vi "GenerateCode.vi"(0 "XRef":T10, 1 "Terms":T7, 2 "Diagram":T6, 3 "State In":T1) -> (14 "Generated Code?":T5, 15 "Reply":T3, 16 "Fatal Error Out":T2, 17 "State Out":T1)   [LabVIEW 2015, in "Set Object Parameters.xnode"]
uses:
  Set Object Parameters.xnode
  <vilib>/XNodeSupport/XNodeXNodeRef.ctl
  <vilib>/XNodeSupport/XNodeTermIDPairs.ctl
  <vilib>/XNodeSupport/XNodeTermIDPair.ctl
  <vilib>/XNodeSupport/XNodeTermRef.ctl
  <vilib>/XNodeSupport/XNodeString.ctl
  <vilib>/XNodeSupport/XNodeTopLevelDiagramRef.ctl
  State.ctl
  <vilib>/XNodeSupport/XNodeBool.ctl
  <vilib>/XNodeSupport/XNodeStringArray.ctl
  <vilib>/XNodeSupport/XNodeErrorCluster.ctl
  <vilib>/Utility/miscctls.llb/LVPointTypeDef.ctl
  Insert Key Value Pair.vi
  <vilib>/XNodeSupport/NI_XNodeSupport.lvlib
  JSON Object.lvclass
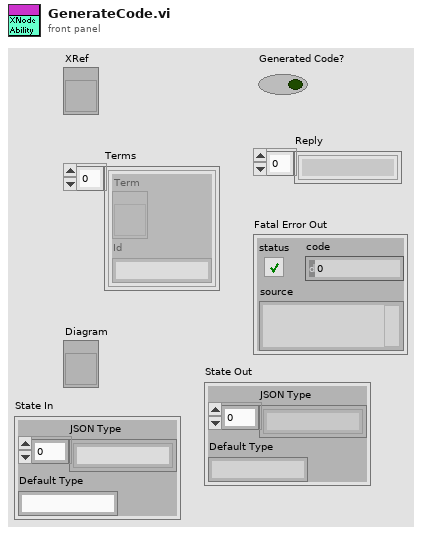
[diagram p1: front panel]
types:
  T1 = typedef "Set Object Parameters.xnode/State.ctl" = cluster{"JSON Type":string[], "Default Type":string}
  T2 = typedef "NI_XNodeSupport.lvlib/XNodeErrorCluster.ctl" = errorcluster
  T3 = typedef "NI_XNodeSupport.lvlib/XNodeStringArray.ctl" = T4[]
  T4 = typedef "NI_XNodeSupport.lvlib/XNodeString.ctl" = string
  T5 = typedef "NI_XNodeSupport.lvlib/XNodeBool.ctl" = bool
  T6 = typedef "NI_XNodeSupport.lvlib/XNodeTopLevelDiagramRef.ctl" = refnum<vi>
  T7 = typedef "NI_XNodeSupport.lvlib/XNodeTermIDPairs.ctl" = T8[]
  T8 = typedef "NI_XNodeSupport.lvlib/XNodeTermIDPair.ctl" = cluster{"Term":T9, "Id":T4}
  T9 = typedef "NI_XNodeSupport.lvlib/XNodeTermRef.ctl" = refnum<vi>
  T10 = typedef "NI_XNodeSupport.lvlib/XNodeXNodeRef.ctl" = refnum<vi>
  T11 = typedef "LVPointTypeDef.ctl" = cluster{"Horizontal":i16, "Vertical":i16}
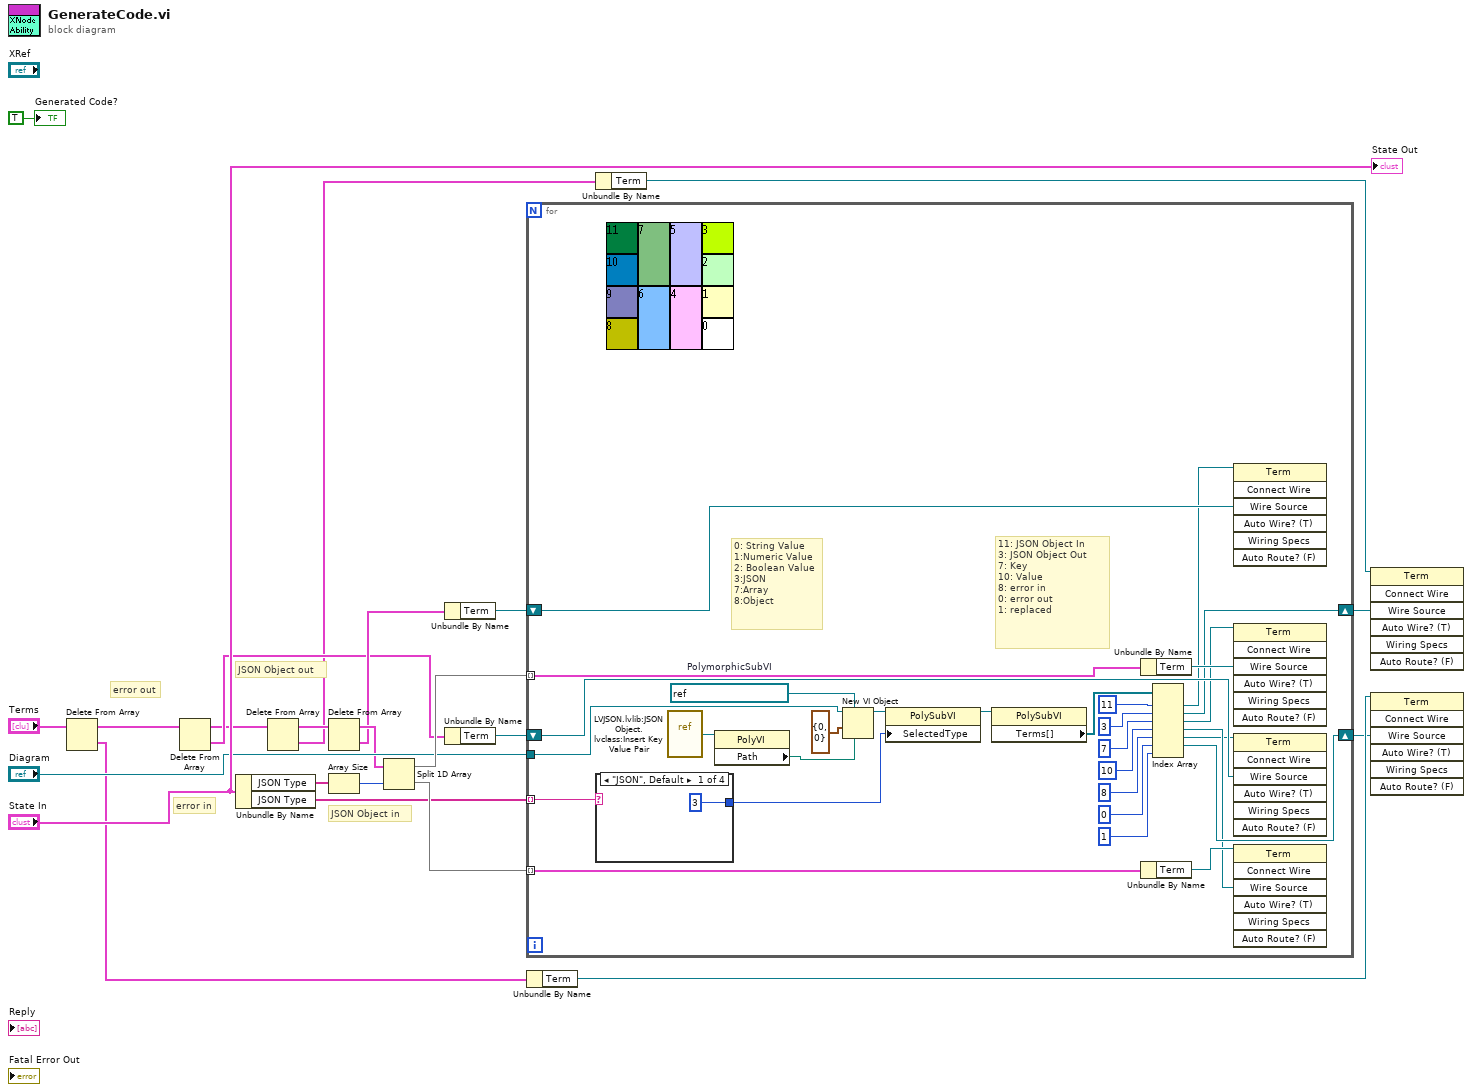
[diagram p0: block diagram]
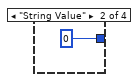
[diagram p2: hidden frame]
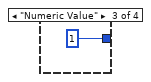
[diagram p3: hidden frame]
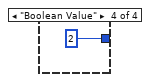
[diagram p4: hidden frame]
diagram:
  # "JSON Object out"
  # "JSON Object in"
  # "error in"
  # "error out"
  n1 = Delete From Array(array="Terms") -> (deleted portion=w12:T8, array with subset deleted=w13:T7)  [unwired: 2 in]
  n2 = Delete From Array(array=w13) -> (deleted portion=w11:T8, array with subset deleted=w5:T7)  [unwired: 2 in]
  n3 = Unbundle By Name("State In") -> ("JSON Type"=w7:string[], "JSON Type"=w15:string[])
  n4 = Delete From Array(array=w5) -> (deleted portion=w3:T8, array with subset deleted=w4:T7)  [unwired: 2 in]
  n5 = Delete From Array(array=w4) -> (deleted portion=w17:T8, array with subset deleted=w18:T7)  [unwired: 2 in]
  n6 = Array Size(array=w7) -> (size(s)=w6:i32)
  n7 = Split 1D Array(array=w18, index=w6) -> (first subarray=w21:T7, second subarray=w20:T7)
  n8 = Unbundle By Name(w17) -> ("Term"=w16:T9)
  n9 = Unbundle By Name(w11) -> ("Term"=w10:T9)
  n10 = for {
    tunnel: w21 -> [w51] mode=indexing
    tunnel: w20 -> [w52] mode=indexing
    tunnel: "Diagram" -> [w47]
    tunnel: w15 -> [w50] mode=indexing
    shift-right: [w27] -> w8
    shift-left: w10 -> [w46]
    shift-right: [w28] -> w1
    shift-left: w16 -> [w45]
    w40 = refnum<vi> refnum  # PolymorphicSubVI
    # "0: String Value\n1:Numeric Value\n2: Boolean Value\n3:JSON\n7:Array\n8:Object"
    # "11: JSON Object In\n3: JSON Object Out\n7: Key\n10: Value\n8: error in\n0: error out\n1: replaced"
    n11 = case shown="\"JSON\", Default" w50 {
      tunnel: [3 ("Selected Type") 0 ("Selected Type") 1 ("Selected Type") 2 ("Selected Type")] -> w48
      frame "JSON", Default {
      }
      frame "String Value" {
      }
      frame "Numeric Value" {
      }
      frame "Boolean Value" {
      }
    }
    n12 = vi-ref "LVJSON.lvlib:JSON Object.lvclass:Insert Key Value Pair.vi"() -> (w37:refnum<vi>)
    n13 = property class="PolyVI"(reference=w37) -> ("Path"=w39:path)  [unwired: 1 in, 2 out]
    n14 = New VI Object(vi object class=w40, owner refnum=w47, position/next to=T11 {"Horizontal"=0, "Vertical"=0} ("location"), 6:w39) -> (object refnum=w38:refnum<vi>)  [unwired: 4 in, 1 out]
    n15 = property class="PolySubVI"(reference=w38, "SelectedType"=w48) -> (reference out=w42:refnum<vi>)  [unwired: 1 in, 1 out]
    n16 = property class="PolySubVI"(reference=w42) -> ("Terms[]"=w43:refnum<vi>[])  [unwired: 1 in, 2 out]
    n17 = Unbundle By Name(w51) -> ("Term"=w33:T9)
    n18 = Unbundle By Name(w52) -> ("Term"=w49:T9)
    n19 = Index Array(array=w43, index #1=11 ("index"), index #2=3 ("index"), index #3=7 ("index"), index #4=10 ("index"), index #5=8 ("index"), index #6=0 ("index"), index #7=1 ("index")) -> (element #1=w29:refnum<vi>, element #2=w28:refnum<vi>, element #3=w26:refnum<vi>, element #4=w25:refnum<vi>, element #5=w24:refnum<vi>, element #6=w27:refnum<vi>)  [unwired: 1 out]
    n20 = invoke class="Term" method="Connect Wire"(reference=w29, "Wire Source"=w45) -> ()  [unwired: 5 in, 7 out]
    n21 = invoke class="Term" method="Connect Wire"(reference=w26, "Wire Source"=w33) -> ()  [unwired: 5 in, 7 out]
    n22 = invoke class="Term" method="Connect Wire"(reference=w24, "Wire Source"=w46) -> ()  [unwired: 5 in, 7 out]
    n23 = invoke class="Term" method="Connect Wire"(reference=w49, "Wire Source"=w25) -> ()  [unwired: 5 in, 7 out]
  }
  n24 = Unbundle By Name(w12) -> ("Term"=w9:T9)
  n25 = Unbundle By Name(w3) -> ("Term"=w2:T9)
  n26 = invoke class="Term" method="Connect Wire"(reference=w2, "Wire Source"=w1) -> ()  [unwired: 5 in, 7 out]
  n27 = invoke class="Term" method="Connect Wire"(reference=w9, "Wire Source"=w8) -> ()  [unwired: 5 in, 7 out]
  "Generated Code?" <- T5 TRUE ("Generated Code?")
  "State Out" <- "State In"
